vi "libssh2_session_callback_set2.vi"(8 "error in (no error)":errorcluster, 9 "callback (0 = use built-in)":u64, 10 "callback type":T1, 11 "session":T2) -> (0 "error out":errorcluster, 2 "previous callback":u64)   [LabVIEW 2017, in "libssh2.lvlib"]
doc: "Set a callback handler for a session. Callbacks are triggered by the receipt of special packets at the transport layer.\n\nSet <B>callback</B> to 0 to to use the built-in default callback handler of lvssh2 (only available when the extension library is enabled). When the extension library is disabled, setting <B>callback</B> to 0 will disable the callback handler."
uses:
  libssh2.lvlib
  Session Refnum.ctl
  libssh2_session_callback_type.ctl
  Not A Session.vi
  <vilib>/Utility/error.llb/Error Cluster From Error Code.vi
  Global Settings.vi
  Read Session Refnum.vi
  <vilib>/Utility/semaphor.llb/Acquire Semaphore.vi
  <vilib>/Utility/semaphor.llb/Release Semaphore.vi
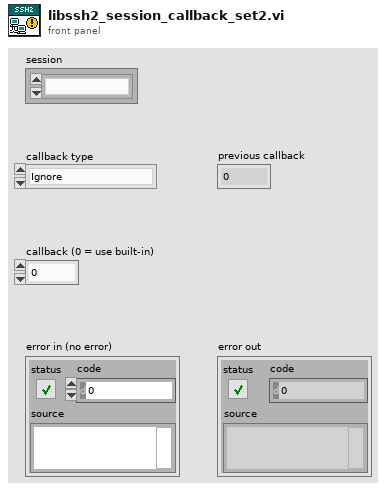
[diagram p1: front panel]
types:
  T1 = typedef "libssh2.lvlib/libssh2_session_callback_type.ctl" = enum16{"Ignore", "Debug", "Disconnect", "MAC Error", "X11", "Send", "Receive", "Auth Agent", "Auth Agent Identities", "Auth Agent Sign"}
  T2 = typedef "libssh2.lvlib/Session Refnum.ctl" = refnum<k1>
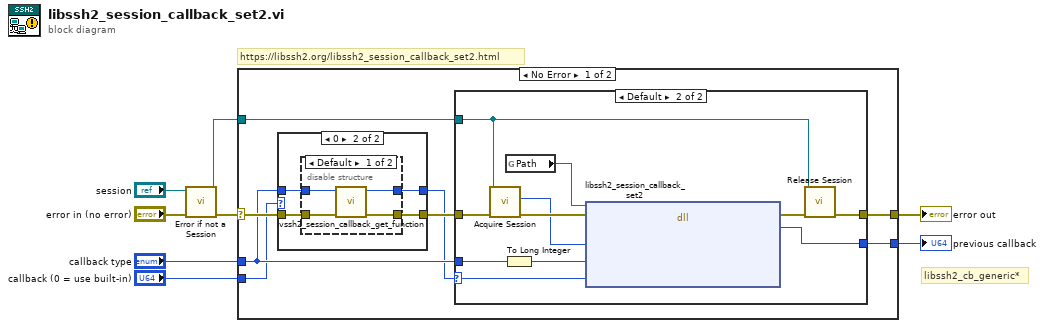
[diagram p0: block diagram]
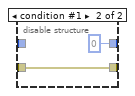
[diagram p4: hidden frame]
diagram:
  # "libssh2_cb_generic*"
  # "https://libssh2.org/libssh2_session_callback_set2.html"
  n1 = call "Error if not a Session.vi"("error in (no error)"="error in (no error)", "session"="session") -> ("error out"=w3:errorcluster, "session out"=w2:T2)  [unwired: 8 in]
  n2 = case shown="No Error" w3 {
    selector: w3 -> [w16 w41]
    tunnel: [w10 w41] -> w8
    tunnel: w2 -> [w9 _]
    tunnel: "callback type" -> [w14 _]
    tunnel: [w13 _] -> w5
    tunnel: "callback (0 = use built-in)" -> [w11 _]
    frame No Error {
      n3 = case shown="0" w11 {
        selector: w11 -> [w30 _]
        tunnel: w16 -> [w29 w34]
        tunnel: [w29 w33] -> w15
        tunnel: w14 -> [_ w32]
        tunnel: [w30 w31] -> w12
        frame Default {
        }
        frame 0 {
          n4 = disable-structure shown="Default" {
            disable-tunnel: w34 -> [w38 w40]
            disable-tunnel: [w37 w40] -> w33
            disable-tunnel: w32 -> [w36 _]
            disable-tunnel: [w35 u64 0 ("callback function")] -> w31
            frame condition #0 (active) {
              n5 = call "lvssh2_session_callback_get_function.vi"("error in (no error)"=w38, "callback type"=w36) -> ("error out"=w37:errorcluster, "callback function"=w35:u64)  [unwired: 8 in]
            }
            frame condition #1 {
            }
          }
        }
      }
      n6 = case shown="Default" w12 {
        selector: w12 -> [_ w20]
        tunnel: w15 -> [w17 w24]
        tunnel: w14 -> [_ w23]
        tunnel: [_ w21] -> w13
        tunnel: [w17 w19] -> w10
        tunnel: w9 -> [_ w18]
        frame 0 {
        }
        frame Default {
          n7 = call "Acquire Session.vi"("error in (no error)"=w24, "session"=w18) -> ("error out"=w28:errorcluster, "LIBSSH2_SESSION*"=w27:u64)  [unwired: 7 in, 1 out]
          n8 = To Long Integer(number=w23) -> (32bit integer=w25:i32)
          n9 = global read "Global Settings.vi" "Path"() -> (w26:path)
          n10 = dll-call lib="?" fn="libssh2_session_callback_set2"(path in=w26, error in=w28, "session"=w27, "cbtype"=w25, "callback"=w20) -> (error out=w22:errorcluster, "return value"=w21:u64)  [unwired: 4 in, 1 out]
          n11 = call "Release Session.vi"("error in (no error)"=w22, "session"=w18) -> ("error out"=w19:errorcluster)  [unwired: 9 in]
        }
      }
    }
    frame Error {
    }
  }
  "error out" <- w8
  "previous callback" <- w5
